vi "Array-Circular Subarray (2D).vi"(8 "Npts":i32, 9 "Offset (in)":i32, 11 "Array":dbl[][](array[numeric])) -> (1 "Offset (out)":i32, 2 "Subarray":dbl[][](array[numeric]))   [LabVIEW 2020]
uses:
  Array-Dimensions (2D).vi
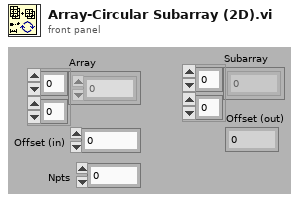
[diagram p1: front panel]
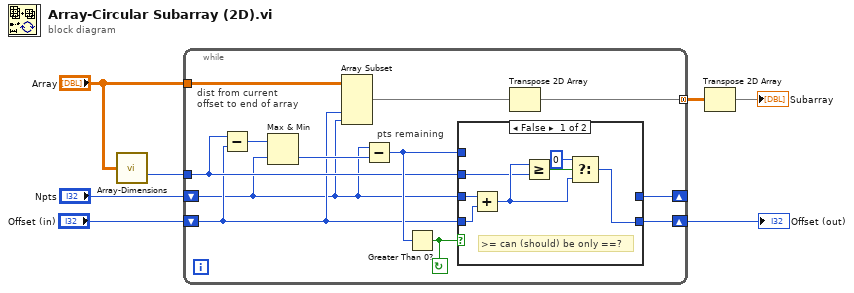
[diagram p0: block diagram]
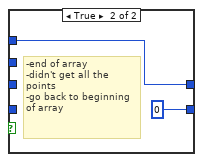
[diagram p2: hidden frame]
diagram:
  n1 = call-poly "Array-Dimensions.vi"("2D Array"="Array") -> ("# columns"=w2:i32)  [unwired: 13 in, 1 out]
  n2 = while {
    tunnel: "Array" -> [w19]
    tunnel: [w8] -> w6 mode=concatenating
    tunnel: w2 -> [w11]
    shift-right: [w12] -> w3
    shift-left: "Offset (in)" -> [w10]
    shift-right: [w14] -> _
    shift-left: "Npts" -> [w9]
    stop <- w15 continue-if-true
    # "pts remaining"
    # "dist from current offset to end of array"
    n3 = Subtract(x=w11, y=w10) -> (x-y=w17:i32)
    n4 = Max & Min(x=w17, y=w9) -> (min(x,y)=w18:i32)  [unwired: 1 out]
    n5 = Array Subset(array=w19, index (col)=w10, length (col)=w9) -> (w13:dbl[][])  [unwired: 2 in]
    n6 = Subtract(x=w9, y=w18) -> (x-y=w16:i32)
    n7 = Greater Than 0?(x=w16) -> (x > 0?=w15:bool)
    n8 = case shown="False" w15 {
      tunnel: w16 -> [_ w28]
      tunnel: w9 -> [w26 _]
      tunnel: w10 -> [w25 _]
      tunnel: [_ w28] -> w14
      tunnel: [w21 0] -> w12
      tunnel: w11 -> [w20 _]
      frame False {
        # ">= can (should) be only ==?"
        n9 = Add(x=w26, y=w25) -> (x+y=w22:i32)
        n10 = Greater Or Equal?(x=w22, y=w20) -> (x >= y?=w24:bool)
        n11 = Select(t=0, s=w24, f=w22) -> (s? t:f=w21:i32)
      }
      frame True {
        # "-end of array\n-didn't get all the points\n-go back to beginning of array"
      }
    }
    n12 = Transpose 2D Array(2D array=w13) -> (transposed array=w8:dbl[][])
  }
  "Offset (out)" <- w3
  n13 = Transpose 2D Array(2D array=w6) -> (transposed array=→"Subarray":dbl[][])
